vi "Handle Drain.vi"(8 "error in (no error)":errorcluster, 11 "Stand in":refnum<class "Stand.lvclass">) -> (0 "error out":errorcluster, 3 "Stand out":refnum<class "Stand.lvclass">)   [LabVIEW 2019, in "Stand.lvclass"]
uses:
  Stand.lvclass
  D:/GIT H4000/H4000/src/Device_class/Device.lvclass
  Stand.lvclass/Stand.ctl
  TypeDef/Mode.ctl
  NeedleValve_class/Cmd.ctl
  Valve Mode.ctl
  Device_class/Device.lvclass/Device.ctl
  Valve State Mode.vi
  Valve State Mode.vi/810e184e-eeb6-4027-a8ae-1422f3ce3d45.vi
  Valve State Mode.vi/57bd4a65-f3dc-44f5-8d68-677c2a197570.vi
  Valve State Mode.vi/03b2f9e4-fceb-4725-9b90-3fd10082a088.vi
  Valve State Mode.vi/2785bab5-dd59-4d13-b638-b9157202fa4a.vi
  Valve State Mode.vi/50faa4b8-a9b4-4cc6-ab66-55c42b424fcd.vi
  Valve State Mode.vi/c882c3fe-b7a7-4419-8f9b-6788aa23338b.vi
  Valve State Mode.vi/3d0d09bd-48e8-482f-b1e2-a36b2bb65234.vi
  Valve State Mode.vi/33d3f26a-dc4a-4f56-bf0a-61d04c5d7434.vi
  Valve State Mode.vi/52af9d47-24d1-4057-80bf-8d93bfb3d17d.vi
  Valve State Mode.vi/bbc9916c-129f-4456-975e-9c3ae3d5db66.vi
  Valve State Mode.vi/a6106d78-2bf9-477e-b655-d47fad07ddfe.vi
  Valve State Mode.vi/e2916439-03c6-4471-bb40-42242a636e27.vi
  Valve State Mode.vi/094228cb-a119-423c-9af8-5a16f059a318.vi
  Valve State Mode.vi/bf5ad1e6-a0ae-4579-ad74-ca8f304cb7cf.vi
  Valve State Mode.vi/eb4d2b76-f0f0-4e1d-bda0-609c5f37b4e7.vi
  Const All Valve.vi
  FPGA_API_class/FPGA API.lvclass
  NeedleValve_class/NeedleValve.lvclass
  PM_Group_class/PM_Group.lvclass
  Device_class/Device.lvclass
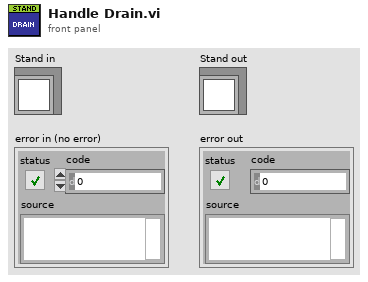
[diagram p1: front panel]
types:
  T1 = typedef "Mode.ctl" = enum16{"IDLE", "FILLING", "EXECUTE_SP", "DRAIN"}
  T2 = typedef "NeedleValve.lvclass/Cmd.ctl" = enum16{"Open", "Close", "Stop"}
  T3 = typedef "Valve Mode.ctl" = enum16{"Filling DUT", "Filling Chamber", "Pump Pressure DUT", "Pump Pressure Chamber", "Haskel Pressure DUT", "Haskel Pressure Chamber", "Slow Release DUT", "Slow Release Chamber", "Fast Release DUT", "Fast Release Chamber", "Fast Release DUT and Chamber", "Leak Pressure DUT", "Leak Pressure Chamber", "Back Pressure DUT", "Back Pressure Chamber", "Fully Closed", "Drain", "Block DUT", "Block Chamber", "filling dut down", "filling chamber down"}
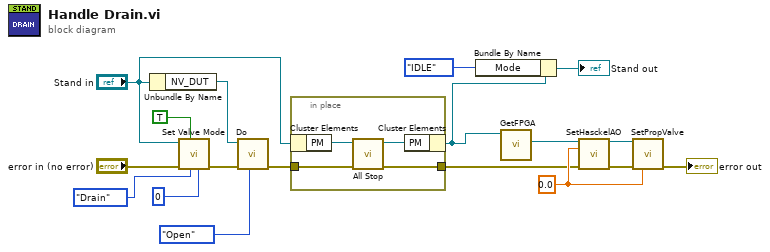
[diagram p0: block diagram]
diagram:
  w6 = 0.0 ("Haskel in")
  n1 = Unbundle By Name("Stand in") -> ("NV_DUT"=w14:refnum<class "NeedleValve.lvclass">)
  n2 = call "Set Valve Mode.vi"("time after close"=u32 0, "Valve DIR"=Valve_Mode."Drain", "init"=TRUE, "error in (no error)"="error in (no error)", "Stand in"="Stand in") -> ("error out"=w13:errorcluster)  [unwired: 5 in, 1 out]
  n3 = call "Do.vi"("Cmd"=Cmd."Open", "error in (no error)"=w13, "NeedleValve in"=w14) -> ("error out"=w10:errorcluster)  [unwired: 7 in, 1 out]
  n4 = in-place {
    in-place-border: w10 -> [w22]
    in-place-border: [w19] -> w4
    n5 = in-place-cluster #1("Stand in") -> ("PM"=w21:refnum<class "PM_Group.lvclass">)
    n6 = call "All Stop.vi"("error in (no error)"=w22, "PM_Group in"=w21) -> ("error out"=w19:errorcluster, "PM_Group out"=w20:refnum<class "PM_Group.lvclass">)  [unwired: 8 in]
    n7 = in-place-cluster #1("PM"=w20) -> (w5:refnum<class "Stand.lvclass">)
  }
  n8 = Bundle By Name(cluster=w5, "Mode"=Mode."IDLE" ("Data.Mode")) -> (→"Stand out":refnum<class "Stand.lvclass">)
  n9 = call "GetFPGA.vi"("Device in"=w5) -> ("FPGA API.lvclass"=w7:refnum<class "FPGA API.lvclass">)  [unwired: 10 in]
  n10 = call-dynamic "SetHasckelAO.vi"("FPGA API in"=w7, "Haskel in"=w6, "error in (no error)"=w4) -> ("FPGA API out"=w9:refnum<class "FPGA API.lvclass">, "error out"=w8:errorcluster)  [unwired: 11 in]
  n11 = call-dynamic "SetPropValve.vi"("FPGA API in"=w9, "error in (no error)"=w8, "AO 1"=w6) -> ("error out"=→"error out":errorcluster)  [unwired: 11 in, 1 out]
